vi "compare_T1_&_T2.vi"(2 "T1":dbl format="%#_13g", 3 "T2":dbl format="%#_13g") -> (7 "Result":enum16{"T1>T2", "T1=T2", "T1<T2"}(ring))   [LabVIEW 2015]
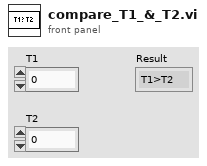
[diagram p1: front panel]
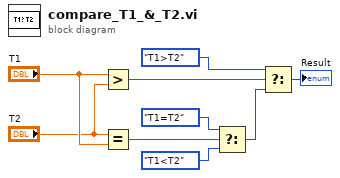
[diagram p0: block diagram]
diagram:
  n1 = Greater?(x="T1", y="T2") -> (0:w1:bool)
  n2 = Equal?(x="T2", y="T1") -> (x = y?=w5:bool)
  n3 = Select(t=enum16{"T1>T2", "T1=T2", "T1<T2"}."T1=T2", s=w5, f=enum16{"T1>T2", "T1=T2", "T1<T2"}."T1<T2") -> (s? t:f=w7:enum16{"T1>T2", "T1=T2", "T1<T2"})
  n4 = Select(t=enum16{"T1>T2", "T1=T2", "T1<T2"}."T1>T2", s=w1, f=w7) -> (s? t:f=→"Result":enum16{"T1>T2", "T1=T2", "T1<T2"})
